vi "Compare file size of FTP to Dir on local Machine.vi"(8 "File Pattern (*.CSV .ddf)":string, 9 "Local Path to compare file sizes to FTP":path, 11 "FTP Creds":T1={"Host"="", "UserName"="", "PassWord"="", "FTP File Path"="", "Timeout (S)"=0, "ActivePasive"=FALSE, "Binary Ascii"=FALSE, "Remote Port"=21} {"Timeout (S)" min=0 max=300 step=1}) -> (3 "Equal File Sizes":cluster{"name":string, "Equal File size":bool}[](array[cluster]))   [LabVIEW 2012]
uses:
  Controls/FTP Credintials.ctl
  <vilib>/FTP/NI_FTP.lvlib
panel:
  in  "Archive Location":path=path "C:/Archive" caption="Directory To Archive *.RAT files"
  # "Passive"
  # "Active"
  # "Binary"
  # "Ascii"
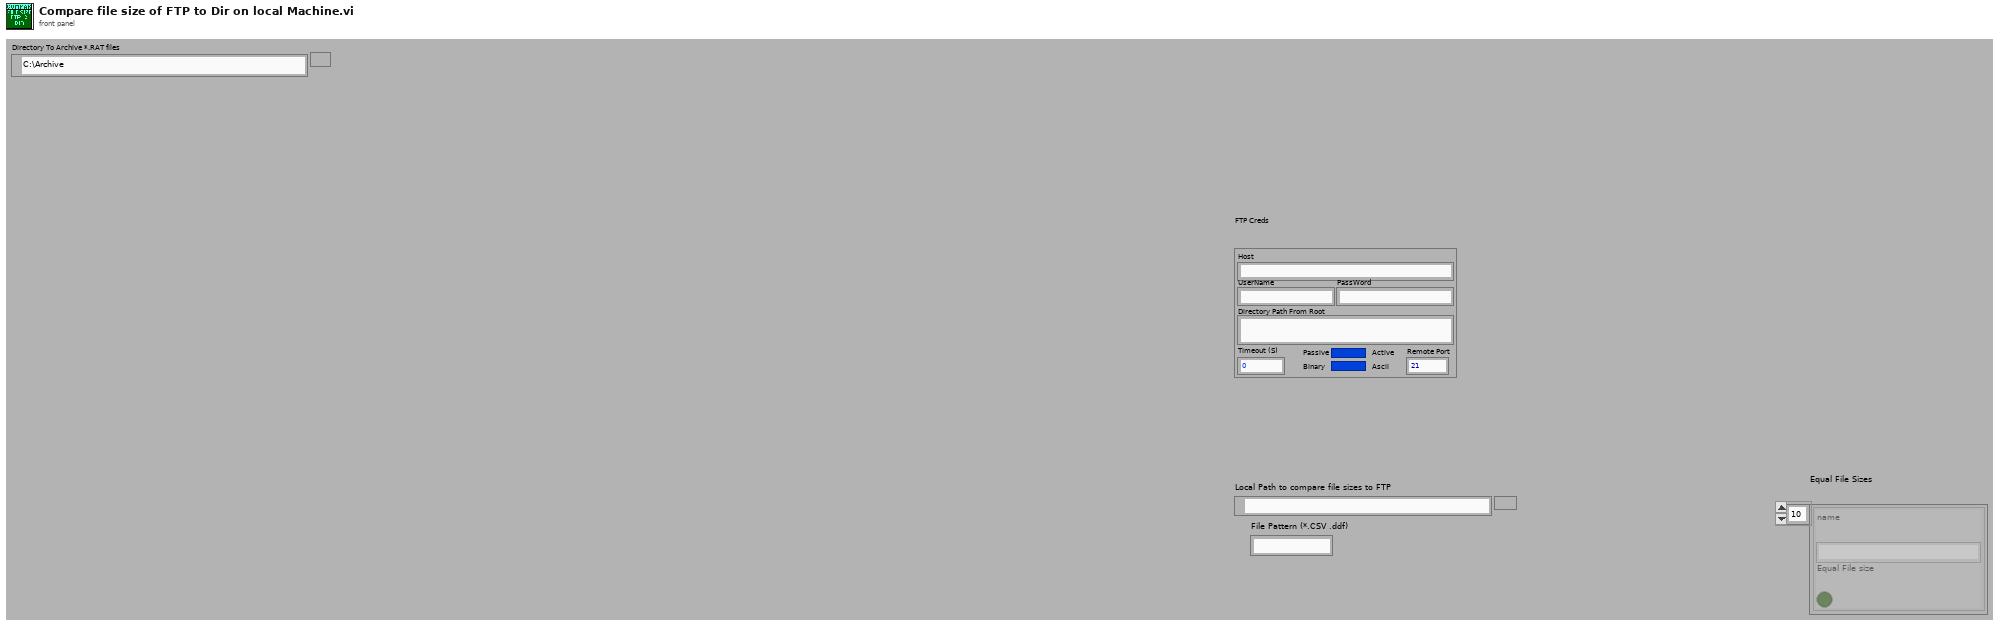
[diagram p1: front panel]
types:
  T1 = typedef "FTP Credintials.ctl" = cluster{"Host":string, "UserName":string, "PassWord":string, "FTP File Path":string, "Timeout (S)":i32, "ActivePasive":bool, "Binary Ascii":bool, "Remote Port":u16}
  T2 = typedef "NI_FTP.lvlib/FTP Session.ctl" = refnum<k5>
  T3 = typedef "NI_FTP.lvlib/FTP File Info.ctl" = cluster{"type":enum16{"unknown", "file", "dir", "link"}, "permissions":string, "owner":string, "group":string, "size":i32, "date":string, "name":string, "link name":string}
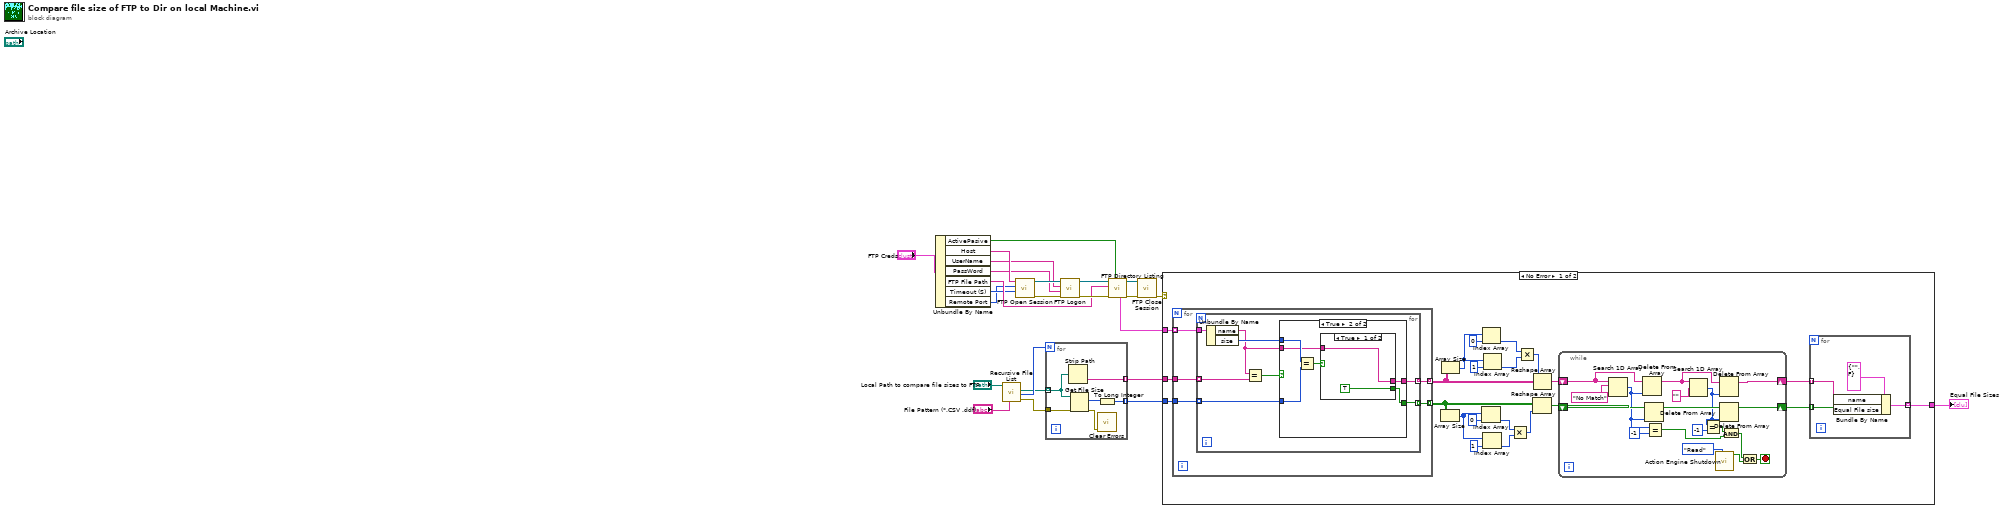
[diagram p0: block diagram]
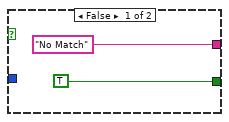
[diagram p2: hidden frame]
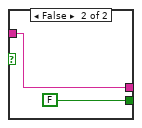
[diagram p3: hidden frame]
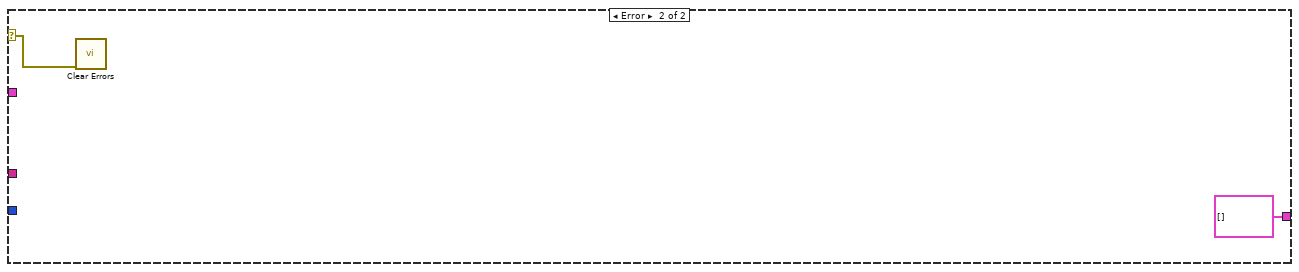
[diagram p4: hidden frame]
diagram:
  n1 = Unbundle By Name("FTP Creds") -> ("ActivePasive"=w6:bool, "Host"=w17:string, "UserName"=w16:string, "PassWord"=w15:string, "FTP File Path"=w14:string, "Timeout (S)"=w3:i32, "Remote Port"=w1:u16)
  n2 = call <vilib>:"Recursive File List.vi"("pattern"="File Pattern (*.CSV .ddf)", "Folder Path"="Local Path to compare file sizes to FTP") -> ("error out"=w2:errorcluster, "Number of Files"=w13:i32, "All Files in Dir"=w12:path[])  [unwired: 5 in, 2 out]
  n3 = call <vilib>:"FTP Open Session.vi"("timeout ms (60000)"=w3, "remote port (21)"=w1, "address"=w17) -> ("error out"=w23:errorcluster, "ftp session"=w24:T2)  [unwired: 5 in, 2 out]
  n4 = for {
    N: w13 -> [_]
    tunnel: w12 -> [w30] mode=indexing
    tunnel: [w29] -> w9 mode=indexing
    tunnel: [w27] -> w8 mode=indexing
    tunnel: w2 -> [w26]
    n5 = Strip Path(path=w30) -> (name=w29:string)  [unwired: 1 out]
    n6 = Get File Size(file=w30, error in=w26) -> (size (in bytes)=w28:i64, 0:w25:errorcluster)  [unwired: 1 out]
    n7 = To Long Integer(number=w28) -> (32bit integer=w27:i32)
    n8 = call <vilib>:"Clear Errors.vi"("error in (no error)"=w25) -> ()  [unwired: 6 in, 1 out]
  }
  n9 = call <vilib>:"FTP Logon.vi"("error in (no error)"=w23, "password"=w15, "user"=w16, "ftp session"=w24) -> ("error out"=w21:errorcluster, "ftp session out"=w22:T2)  [unwired: 4 in, 2 out]
  n10 = call <vilib>:"FTP Directory Listing.vi"("active (T)"=w6, "error in (no error)"=w21, "directory path"=w14, "ftp session"=w22) -> ("error out"=w19:errorcluster, "ftp session out"=w20:T2, "dir list"=w10:T3[])  [unwired: 3 in, 2 out]
  n11 = call <vilib>:"FTP Close Session.vi"("error in (no error)"=w19, "ftp session"=w20) -> ("error out"=w4:errorcluster)  [unwired: 6 in, 3 out]
  n12 = case shown="No Error" w4 {
    selector: w4 -> [_ w101]
    tunnel: w10 -> [w52 _]
    tunnel: w9 -> [w51 _]
    tunnel: w8 -> [w50 _]
    tunnel: [w47 cluster{"name":string, "Equal File size":bool}[] []] -> w7
    frame No Error {
      n13 = for {
        tunnel: w52 -> [w79] mode=indexing
        tunnel: w51 -> [w78]
        tunnel: w50 -> [w77]
        tunnel: [w76] -> w33 mode=indexing
        tunnel: [w75] -> w46 mode=indexing
        n14 = for {
          tunnel: w79 -> [w87]
          tunnel: w78 -> [w85] mode=indexing
          tunnel: w77 -> [w83] mode=indexing
          tunnel: [w81] -> w75 mode=indexing
          tunnel: [w80] -> w76 mode=indexing
          n15 = Unbundle By Name(w87) -> ("name"=w82:string, "size"=w84:i32)
          n16 = Equal?(x=w82, y=w85) -> (x = y?=w86:bool)
          n17 = case shown="True" w86 {
            tunnel: w84 -> [_ w94]
            tunnel: w83 -> [_ w93]
            tunnel: w82 -> [_ w92]
            tunnel: ["No Match" ("name") w90] -> w81
            tunnel: [TRUE w91] -> w80
            frame False {
            }
            frame True {
              n18 = Equal?(x=w94, y=w93) -> (x = y?=w95:bool)
              n19 = case shown="True" w95 {
                tunnel: w92 -> [w96 w98]
                tunnel: [TRUE FALSE] -> w91
                tunnel: [w96 w98] -> w90
                frame True {
                }
                frame False {
                }
              }
            }
          }
        }
      }
      n20 = Array Size(array=w33) -> (size(s)=w36:i32[])
      n21 = Array Size(array=w46) -> (size(s)=w43:i32[])
      n22 = Index Array(array=w36, index=0) -> (element=w37:i32)
      n23 = Index Array(array=w43, index=0) -> (element=w42:i32)
      n24 = Index Array(array=w36, index=1) -> (element=w38:i32)
      n25 = Index Array(array=w43, index=1) -> (element=w41:i32)
      n26 = Multiply(x=w37, y=w38) -> (x*y=w39:i32)
      n27 = Multiply(x=w42, y=w41) -> (x*y=w40:i32)
      n28 = Reshape Array(w33, w39) -> (w31:bool[])
      n29 = Reshape Array(w46, w40) -> (w32:string[])
      n30 = while {
        shift-right: [w66] -> w49
        shift-left: w32 -> [w73]
        shift-right: [w67] -> w48
        shift-left: w31 -> [w72]
        stop <- w60 stop-if-true
        n31 = Search 1D Array(1D array=w73, element="No Match" ("name")) -> (index of element=w71:i32)  [unwired: 1 in]
        n32 = Delete From Array(array=w73, index=w71) -> (array with subset deleted=w65:string[])  [unwired: 1 in, 1 out]
        n33 = Delete From Array(array=w72, index=w71) -> (array with subset deleted=w68:bool[])  [unwired: 1 in, 1 out]
        n34 = Equal?(x=w71, y=-1) -> (x = y?=w61:bool)
        n35 = Search 1D Array(1D array=w65, element="" ("name")) -> (index of element=w63:i32)  [unwired: 1 in]
        n36 = Equal?(x=w63, y=-1) -> (x = y?=w62:bool)
        n37 = call "Action Engine Shutdown.vi"("Shutdown"=enum16{"Write", "Read"}."Read") -> ("Shutdown"=w57:bool)  [unwired: 9 in, 1 out]
        n38 = Delete From Array(array=w65, index=w63) -> (array with subset deleted=w66:string[])  [unwired: 1 in, 1 out]
        n39 = Delete From Array(array=w68, index=w63) -> (array with subset deleted=w67:bool[])  [unwired: 1 in, 1 out]
        n40 = And(x=w62, y=w61) -> (x .and. y?=w59:bool)
        n41 = Or(x=w59, y=w57) -> (x .or. y?=w60:bool)
      }
      n42 = for {
        tunnel: w49 -> [w55] mode=indexing
        tunnel: w48 -> [w54] mode=indexing
        tunnel: [w53] -> w47 mode=indexing
        n43 = Bundle By Name(cluster=cluster{"name":string, "Equal File size":bool} {"name"="", "Equal File size"=FALSE} ("input cluster"), "name"=w55, "Equal File size"=w54) -> (w53:cluster{"name":string, "Equal File size":bool})
      }
    }
    frame Error {
      n44 = call <vilib>:"Clear Errors.vi"("error in (no error)"=w101) -> ()  [unwired: 6 in, 1 out]
    }
  }
  "Equal File Sizes" <- w7
